vi "Input setup for Move birmorph.vi"(5 "AI max value":dbl=10.0 caption="Input Maximum Value" format="%0.2f", 7 "AI min value":dbl=-10.0 caption="Input Minimum Value" format="%0.2f", 10 "Sample rate (Hz)":dbl=1000.0 format="%0.2f", 11 "AI channels":tag="Dev2/ai0:1" caption="Input Physical Channel") -> (0 "error out":errorcluster, 3 "AI task out":refnum<k21>)   [LabVIEW 2010]
uses:
  <vilib>/DAQmx/create/channels.llb/DAQmx Create Channel (AI-Voltage-Basic).vi
  <vilib>/DAQmx/configure/timing.llb/DAQmx Timing (Sample Clock).vi
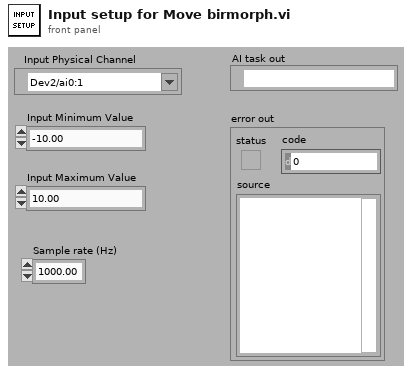
[diagram p1: front panel]
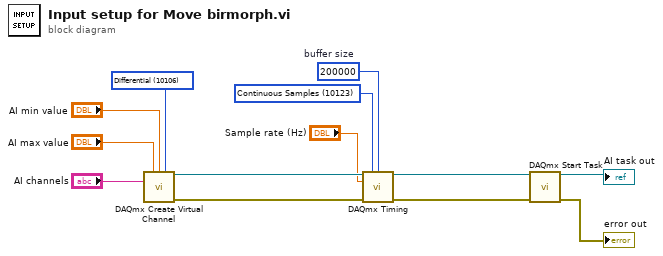
[diagram p0: block diagram]
diagram:
  w4 = 10106 items=["default"=-1, "RSE"=10083, "NRSE"=10078, "Differential"=10106, "Pseudodifferential"=12529] ("input terminal configuration")
  w5 = 200000  # buffer size
  w9 = 10123 items=["Finite Samples"=10178, "Continuous Samples"=10123] ("sample mode")
  n1 = call-poly <vilib>:"DAQmx Create Virtual Channel.vi"("maximum value"="AI max value", "minimum value"="AI min value", "input terminal configuration"=w4, "physical channels"="AI channels") -> ("task out"=w11:refnum<k21>, "error out"=w10:errorcluster)  [unwired: 10 in]
  n2 = call-poly <vilib>:"DAQmx Timing.vi"("task/channels in"=w11, "sample mode"=w9, "samples per channel"=w5, "rate"="Sample rate (Hz)", "error in"=w10) -> ("task out"=w3:refnum<k21>, "error out"=w2:errorcluster)  [unwired: 9 in]
  n3 = call <vilib>:"DAQmx Start Task.vi"("task/channels in"=w3, "error in"=w2) -> ("task out"=→"AI task out":refnum<k21>, "error out"=→"error out":errorcluster)  [unwired: 12 in]
